vi "IsNumeric.vi"(4 "Value String in":string) -> (0 "IsNumeric":bool, 2 "Numeric Value":ext)   [LabVIEW 2016]
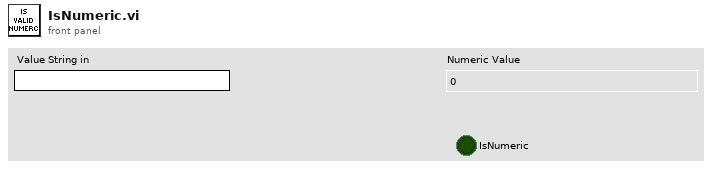
[diagram p1: front panel]
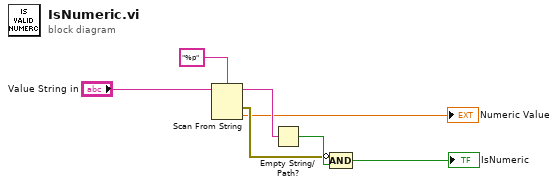
[diagram p0: block diagram]
diagram:
  n1 = Scan From String(format string="%p", input string="Value String in") -> (remaining string=w6:string, error out=w3:errorcluster, output 1=→"Numeric Value":ext)  [unwired: 3 in, 1 out]
  n2 = Empty String/Path?(string/path=w6) -> (empty?=w5:bool)
  n3 = Compound Arithmetic op=AND(invert w3, w5) -> (→"IsNumeric":bool)
